vi "ConvertDecToASCII.vi"(1 "String Decimal":string) -> (0 "String Out":string)   [LabVIEW 2016]
doc: "Recives an Hexadecimal String and converts it to Variant"
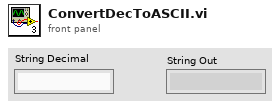
[diagram p1: front panel]
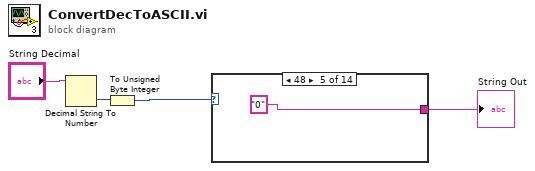
[diagram p0: block diagram]
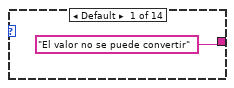
[diagram p2: hidden frame]
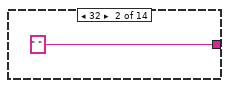
[diagram p3: hidden frame]
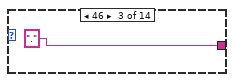
[diagram p4: hidden frame]
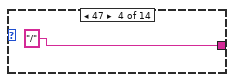
[diagram p5: hidden frame]
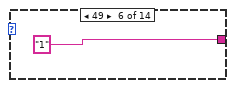
[diagram p6: hidden frame]
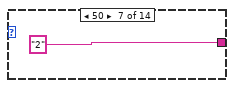
[diagram p7: hidden frame]
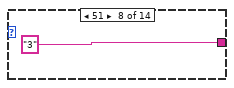
[diagram p8: hidden frame]
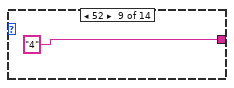
[diagram p9: hidden frame]
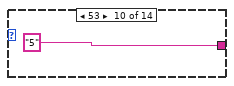
[diagram p10: hidden frame]
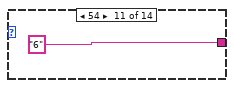
[diagram p11: hidden frame]
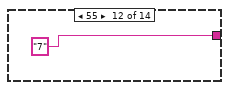
[diagram p12: hidden frame]
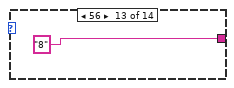
[diagram p13: hidden frame]
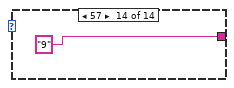
[diagram p14: hidden frame]
diagram:
  n1 = Decimal String To Number(string="String Decimal") -> (number=w2:i32)  [unwired: 2 in, 1 out]
  n2 = To Unsigned Byte Integer(number=w2) -> (unsigned 8bit integer=w4:u8)
  n3 = case shown="48" w4 {
    tunnel: ["El valor no se puede convertir" " " "." "/" "0" "1" "2" "3" "4" "5" "6" "7" "8" "9"] -> w1
    frame Default {
    }
    frame 32 {
    }
    frame 46 {
    }
    frame 47 {
    }
    frame 48 {
    }
    frame 49 {
    }
    frame 50 {
    }
    frame 51 {
    }
    frame 52 {
    }
    frame 53 {
    }
    frame 54 {
    }
    frame 55 {
    }
    frame 56 {
    }
    frame 57 {
    }
  }
  "String Out" <- w1
